vi "test ni-switch.vi"() -> ()   [LabVIEW 2021]
uses:
  <instrlib>/niSwitch/niSwitch.llb/niSwitch Topologies.ctl
panel:
  in  "topology name":T1="Configured Topology" caption="Topology Name"
  in  "relay action":i32(ring)=21 caption="Relay Action" items=["Open Relay"=20, "Close Relay"=21]
  in  "resource name":refnum<k15>="PXI1Slot2" caption="Resource Name"
  in  "relay name":string="k0" caption="Relay Name"
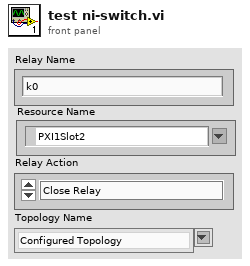
[diagram p1: front panel]
types:
  T1 = typedef "niSwitch Topologies.ctl" = string
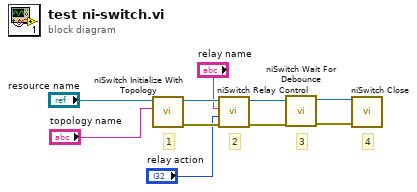
[diagram p0: block diagram]
diagram:
  # "4"
  # "3"
  # "2"
  # "1"
  n1 = call <instrlib>:"niSwitch Initialize With Topology.vi"("topology name"="topology name", "resource name"="resource name") -> ("error out"=w10:errorcluster, "instrument handle out"=w9:refnum<k15>)  [unwired: 3 in, 5 out]
  n2 = call <instrlib>:"niSwitch Relay Control.vi"("error in (no error)"=w10, "relay action (Close Relay)"="relay action", "relay names"="relay name", "instrument handle"=w9) -> ("error out"=w4:errorcluster, "instrument handle out"=w5:refnum<k15>)  [unwired: 6 out]
  n3 = call <instrlib>:"niSwitch Wait For Debounce.vi"("error in (no error)"=w4, "instrument handle"=w5) -> ("error out"=w2:errorcluster, "instrument handle out"=w3:refnum<k15>)  [unwired: 1 in, 7 out]
  n4 = call <instrlib>:"niSwitch Close.vi"("error in (no error)"=w2, "instrument handle"=w3) -> ()  [unwired: 10 out]
